vi "time.vi"() -> ()   [LabVIEW 2018]
panel:
  out "Wait Until Next ms Multiple":u32[](graph)
  out "Time Delay":u32[](graph)
  out "Wait":u32[](graph)
  out "Time Delay":u32[](array[numeric])
  out "Wait Until Next ms Multiple":u32[](array[numeric])
  out "Wait":u32[](array[numeric])
  in  "Time Delay":dbl=1.0 caption="Delay Time (s)"
  in  "Wait Until Next ms Multiple":u32
  in  "Wait":u32
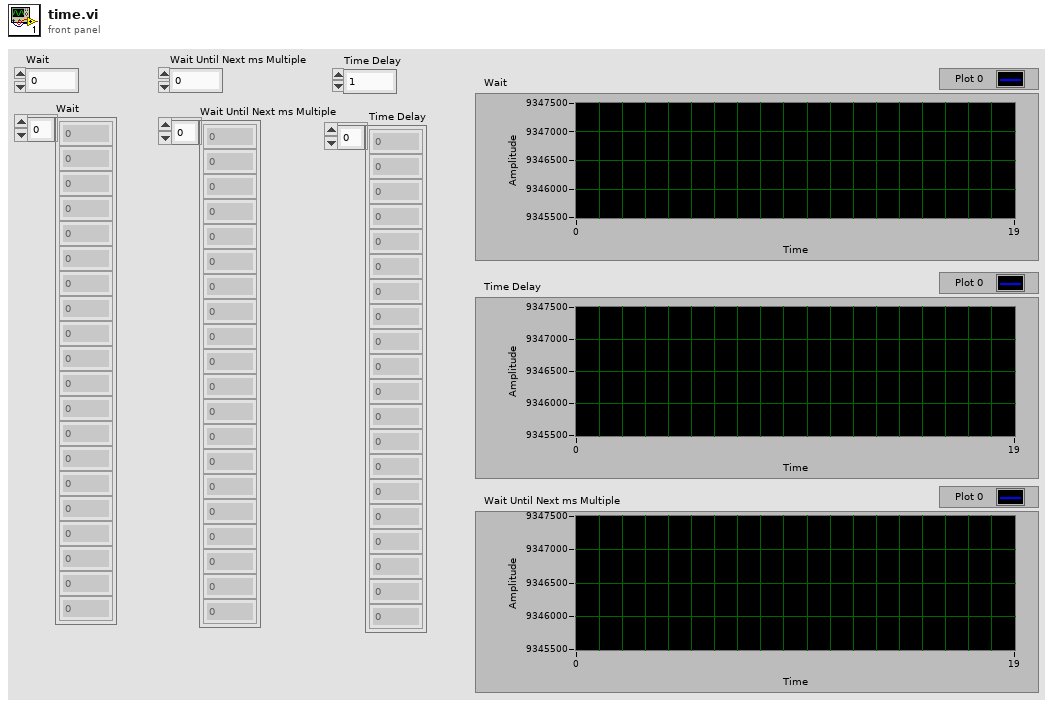
[diagram p1: front panel]
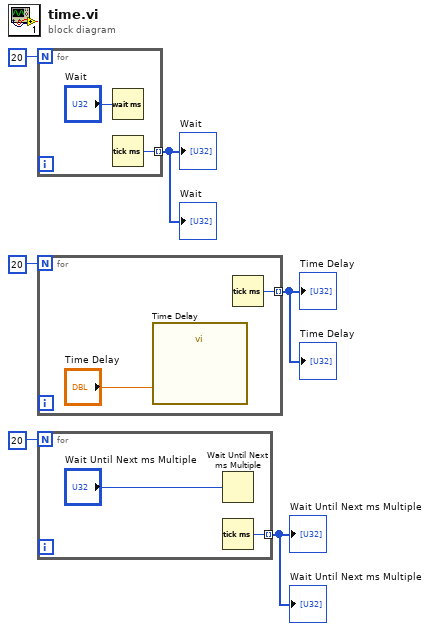
[diagram p0: block diagram]
diagram:
  n1 = for {
    N: 20 -> [_]
    tunnel: [w7] -> w3 mode=indexing
    n2 = Wait (ms)(milliseconds to wait="Wait") -> ()  [unwired: 1 out]
    n3 = Tick Count (ms)() -> (millisecond timer value=w7:u32)
  }
  "Wait" <- w3
  "Wait" <- w3
  n4 = for {
    N: 20 -> [_]
    tunnel: [w9] -> w2 mode=indexing
    n5 = call "Time Delay"("Delay Time (s)"="Time Delay") -> ()  [unwired: 10 in, 1 out]
    n6 = Tick Count (ms)() -> (millisecond timer value=w9:u32)
  }
  "Time Delay" <- w2
  "Time Delay" <- w2
  n7 = for {
    N: 20 -> [_]
    tunnel: [w11] -> w1 mode=indexing
    n8 = Wait Until Next ms Multiple(millisecond multiple="Wait Until Next ms Multiple") -> ()  [unwired: 1 out]
    n9 = Tick Count (ms)() -> (millisecond timer value=w11:u32)
  }
  "Wait Until Next ms Multiple" <- w1
  "Wait Until Next ms Multiple" <- w1
